vi "equipconfirm.vi"(1 "path to XML document":path caption="XML文档路径") -> (0 "确认结果":bool)   [LabVIEW 2011]
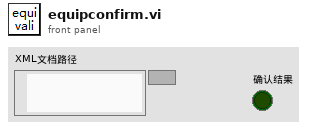
[diagram p1: front panel]
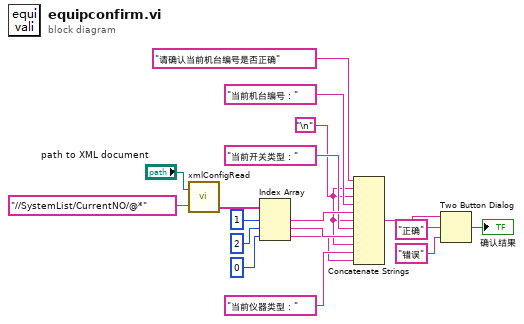
[diagram p0: block diagram]
diagram:
  w1 = "\n"
  n1 = call "xmlConfigRead.vi"("path to XML document"="path to XML document", "XPath expression"="//SystemList/CurrentNO/@*") -> ("OutParaArray"=w16:string[])  [unwired: 2 out]
  n2 = Index Array(array=w16, index #1=1 ("索引"), index #2=2 ("索引"), index #3=0 ("索引")) -> (element #1=w12:string, element #2=w10:string, element #3=w8:string)
  n3 = Concatenate Strings("请确认当前机台编号是否正确" ("字符串"), w1, w1, "当前机台编号：" ("字符串"), w12, w1, "当前开关类型：" ("字符串"), w10, w1, "当前仪器类型：" ("字符串"), w8) -> (w7:string)
  n4 = Two Button Dialog(message=w7, 1:"错误" ("F按钮名称（“取消”）"), 2:"正确" ("T按钮名称（“确定”）")) -> (T button?=→"确认结果":bool)
